vi "FindFaces.vi"   [LabVIEW 2017, in "ImageFacialDetection.lvclass"]
uses:
  ImageFacialDetection.lvclass
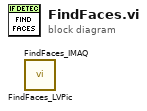
[diagram p0: block diagram]
diagram:
  n1 = call-dynamic "FindFaces_LVPic.vi"() -> ()  [unwired: 9 in, 3 out]
  n2 = call-dynamic "FindFaces_IMAQ.vi"() -> ()  [unwired: 9 in, 3 out]
